vi "EOL All-Station Check Switch Signals.vi"(0 "Current Data In":sgl[][](array[numeric]), 1 "Switch Value Configuration":T3[](array[typedef])=[{"All Motions"=enum."Glass Teach", "Array"=[{"Min"=0.0, "Max"=0.0, "Check?"=FALSE}, {"Min"=0.0, "Max"=0.0, "Check?"=FALSE}, {"Min"=0.0, "Max"=0.0, "Check?"=FALSE}, {"Min"=0.0, "Max"=0.0, "Check?"=FALSE}, {"Min"=0.0, "Max"=0.0, "Check?"=FALSE}, {"Min"=0.0, "Max"=0.0, "Check?"=FALSE}, {"Min"=0.0, "Max"=0.0, "Check?"=FALSE}, {"Min"=0.0, "Max"=0.0, "Check?"=FALSE}, {"Min"=0.0, "Max"=0.0, "Check?"=FALSE}, {"Min"=0.0, "Max"=0.0, "Check?"=FALSE}, {"Min"=0.0, "Max"=0.0, "Check?"=FALSE}]}, {"All Motions"=enum."Glass Slide Open", "Array"=[{"Min"=0.0, "Max"=0.0, "Check?"=FALSE}, {"Min"=0.0, "Max"=0.0, "Check?"=FALSE}, {"Min"=0.0, "Max"=0.0, "Check?"=FALSE}, {"Min"=0.0, "Max"=0.0, "Check?"=FALSE}, {"Min"=0.0, "Max"=0.0, "Check?"=FALSE}, {"Min"=0.0, "Max"=0.0, "Check?"=FALSE}, {"Min"=0.0, "Max"=0.0, "Check?"=FALSE}, {"Min"=0.0, "Max"=0.0, "Check?"=FALSE}, {"Min"=0.0, "Max"=0.0, "Check?"=FALSE}, {"Min"=0.0, "Max"=0.0, "Check?"=FALSE}, {"Min"=0.0, "Max"=0.0, "Check?"=FALSE}]}, {"All Motions"=enum."Glass Slide Close", "Array"=[{"Min"=0.0, "Max"=0.0, "Check?"=FALSE}, {"Min"=0.0, "Max"=0.0, "Check?"=FALSE}, {"Min"=0.0, "Max"=0.0, "Check?"=FALSE}, {"Min"=0.0, "Max"=0.0, "Check?"=FALSE}, {"Min"=0.0, "Max"=0.0, "Check?"=FALSE}, {"Min"=0.0, "Max"=0.0, "Check?"=FALSE}, {"Min"=0.0, "Max"=0.0, "Check?"=FALSE}, {"Min"=0.0, "Max"=0.0, "Check?"=FALSE}, {"Min"=0.0, "Max"=0.0, "Check?"=FALSE}, {"Min"=0.0, "Max"=0.0, "Check?"=FALSE}, {"Min"=0.0, "Max"=0.0, "Check?"=FALSE}]}, {"All Motions"=enum."Glass Vent Open", "Array"=[{"Min"=0.0, "Max"=0.0, "Check?"=FALSE}, {"Min"=0.0, "Max"=0.0, "Check?"=FALSE}, {"Min"=0.0, "Max"=0.0, "Check?"=FALSE}, {"Min"=0.0, "Max"=0.0, "Check?"=FALSE}, {"Min"=0.0, "Max"=0.0, "Check?"=FALSE}, {"Min"=0.0, "Max"=0.0, "Check?"=FALSE}, {"Min"=0.0, "Max"=0.0, "Check?"=FALSE}, {"Min"=0.0, "Max"=0.0, "Check?"=FALSE}, {"Min"=0.0, "Max"=0.0, "Check?"=FALSE}, {"Min"=0.0, "Max"=0.0, "Check?"=FALSE}, {"Min"=0.0, "Max"=0.0, "Check?"=FALSE}]}, {"All Motions"=enum."Sunshade Teach", "Array"=[{"Min"=0.0, "Max"=0.0, "Check?"=FALSE}, {"Min"=0.0, "Max"=0.0, "Check?"=FALSE}, {"Min"=0.0, "Max"=0.0, "Check?"=FALSE}, {"Min"=0.0, "Max"=0.0, "Check?"=FALSE}, {"Min"=0.0, "Max"=0.0, "Check?"=FALSE}, {"Min"=0.0, "Max"=0.0, "Check?"=FALSE}, {"Min"=0.0, "Max"=0.0, "Check?"=FALSE}, {"Min"=0.0, "Max"=0.0, "Check?"=FALSE}, {"Min"=0.0, "Max"=0.0, "Check?"=FALSE}, {"Min"=0.0, "Max"=0.0, "Check?"=FALSE}, {"Min"=0.0, "Max"=0.0, "Check?"=FALSE}]}, {"All Motions"=enum."Sunshade Open", "Array"=[{"Min"=0.0, "Max"=0.0, "Check?"=FALSE}, {"Min"=0.0, "Max"=0.0, "Check?"=FALSE}, {"Min"=0.0, "Max"=0.0, "Check?"=FALSE}, {"Min"=0.0, "Max"=0.0, "Check?"=FALSE}, {"Min"=0.0, "Max"=0.0, "Check?"=FALSE}, {"Min"=0.0, "Max"=0.0, "Check?"=FALSE}, {"Min"=0.0, "Max"=0.0, "Check?"=FALSE}, {"Min"=0.0, "Max"=0.0, "Check?"=FALSE}, {"Min"=0.0, "Max"=0.0, "Check?"=FALSE}, {"Min"=0.0, "Max"=0.0, "Check?"=FALSE}, {"Min"=0.0, "Max"=0.0, "Check?"=FALSE}]}, {"All Motions"=enum."Sunshade Close", "Array"=[{"Min"=0.0, "Max"=0.0, "Check?"=FALSE}, {"Min"=0.0, "Max"=0.0, "Check?"=FALSE}, {"Min"=0.0, "Max"=0.0, "Check?"=FALSE}, {"Min"=0.0, "Max"=0.0, "Check?"=FALSE}, {"Min"=0.0, "Max"=0.0, "Check?"=FALSE}, {"Min"=0.0, "Max"=0.0, "Check?"=FALSE}, {"Min"=0.0, "Max"=0.0, "Check?"=FALSE}, {"Min"=0.0, "Max"=0.0, "Check?"=FALSE}, {"Min"=0.0, "Max"=0.0, "Check?"=FALSE}, {"Min"=0.0, "Max"=0.0, "Check?"=FALSE}, {"Min"=0.0, "Max"=0.0, "Check?"=FALSE}]}, {"All Motions"=enum."Idle", "Array"=[{"Min"=0.0, "Max"=0.0, "Check?"=FALSE}, {"Min"=0.0, "Max"=0.0, "Check?"=FALSE}, {"Min"=0.0, "Max"=0.0, "Check?"=FALSE}, {"Min"=0.0, "Max"=0.0, "Check?"=FALSE}, {"Min"=0.0, "Max"=0.0, "Check?"=FALSE}, {"Min"=0.0, "Max"=0.0, "Check?"=FALSE}, {"Min"=0.0, "Max"=0.0, "Check?"=FALSE}, {"Min"=0.0, "Max"=0.0, "Check?"=FALSE}, {"Min"=0.0, "Max"=0.0, "Check?"=FALSE}, {"Min"=0.0, "Max"=0.0, "Check?"=FALSE}, {"Min"=0.0, "Max"=0.0, "Check?"=FALSE}]}, {"All Motions"=enum."Sunshade Open 2", "Array"=[{"Min"=0.0, "Max"=0.0, "Check?"=FALSE}, {"Min"=0.0, "Max"=0.0, "Check?"=FALSE}, {"Min"=0.0, "Max"=0.0, "Check?"=FALSE}, {"Min"=0.0, "Max"=0.0, "Check?"=FALSE}, {"Min"=0.0, "Max"=0.0, "Check?"=FALSE}, {"Min"=0.0, "Max"=0.0, "Check?"=FALSE}, {"Min"=0.0, "Max"=0.0, "Check?"=FALSE}, {"Min"=0.0, "Max"=0.0, "Check?"=FALSE}, {"Min"=0.0, "Max"=0.0, "Check?"=FALSE}, {"Min"=0.0, "Max"=0.0, "Check?"=FALSE}, {"Min"=0.0, "Max"=0.0, "Check?"=FALSE}]}, {"All Motions"=enum."Sunshade Close 2", "Array"=[{"Min"=0.0, "Max"=0.0, "Check?"=FALSE}, {"Min"=0.0, "Max"=0.0, "Check?"=FALSE}, {"Min"=0.0, "Max"=0.0, "Check?"=FALSE}, {"Min"=0.0, "Max"=0.0, "Check?"=FALSE}, {"Min"=0.0, "Max"=0.0, "Check?"=FALSE}, {"Min"=0.0, "Max"=0.0, "Check?"=FALSE}, {"Min"=0.0, "Max"=0.0, "Check?"=FALSE}, {"Min"=0.0, "Max"=0.0, "Check?"=FALSE}, {"Min"=0.0, "Max"=0.0, "Check?"=FALSE}, {"Min"=0.0, "Max"=0.0, "Check?"=FALSE}, {"Min"=0.0, "Max"=0.0, "Check?"=FALSE}]}, {"All Motions"=enum."Glass Slide Open Sunshade Open", "Array"=[{"Min"=0.0, "Max"=0.0, "Check?"=FALSE}, {"Min"=0.0, "Max"=0.0, "Check?"=FALSE}, {"Min"=0.0, "Max"=0.0, "Check?"=FALSE}, {"Min"=0.0, "Max"=0.0, "Check?"=FALSE}, {"Min"=0.0, "Max"=0.0, "Check?"=FALSE}, {"Min"=0.0, "Max"=0.0, "Check?"=FALSE}, {"Min"=0.0, "Max"=0.0, "Check?"=FALSE}, {"Min"=0.0, "Max"=0.0, "Check?"=FALSE}, {"Min"=0.0, "Max"=0.0, "Check?"=FALSE}, {"Min"=0.0, "Max"=0.0, "Check?"=FALSE}, {"Min"=0.0, "Max"=0.0, "Check?"=FALSE}]}, {"All Motions"=enum."Glass Slide Open Sunshade Close", "Array"=[{"Min"=0.0, "Max"=0.0, "Check?"=FALSE}, {"Min"=0.0, "Max"=0.0, "Check?"=FALSE}, {"Min"=0.0, "Max"=0.0, "Check?"=FALSE}, {"Min"=0.0, "Max"=0.0, "Check?"=FALSE}, {"Min"=0.0, "Max"=0.0, "Check?"=FALSE}, {"Min"=0.0, "Max"=0.0, "Check?"=FALSE}, {"Min"=0.0, "Max"=0.0, "Check?"=FALSE}, {"Min"=0.0, "Max"=0.0, "Check?"=FALSE}, {"Min"=0.0, "Max"=0.0, "Check?"=FALSE}, {"Min"=0.0, "Max"=0.0, "Check?"=FALSE}, {"Min"=0.0, "Max"=0.0, "Check?"=FALSE}]}, {"All Motions"=enum."Glass Slide Close Sunshade Open", "Array"=[{"Min"=0.0, "Max"=0.0, "Check?"=FALSE}, {"Min"=0.0, "Max"=0.0, "Check?"=FALSE}, {"Min"=0.0, "Max"=0.0, "Check?"=FALSE}, {"Min"=0.0, "Max"=0.0, "Check?"=FALSE}, {"Min"=0.0, "Max"=0.0, "Check?"=FALSE}, {"Min"=0.0, "Max"=0.0, "Check?"=FALSE}, {"Min"=0.0, "Max"=0.0, "Check?"=FALSE}, {"Min"=0.0, "Max"=0.0, "Check?"=FALSE}, {"Min"=0.0, "Max"=0.0, "Check?"=FALSE}, {"Min"=0.0, "Max"=0.0, "Check?"=FALSE}, {"Min"=0.0, "Max"=0.0, "Check?"=FALSE}]}, {"All Motions"=enum."Glass Slide Close Sunshade Close", "Array"=[{"Min"=0.0, "Max"=0.0, "Check?"=FALSE}, {"Min"=0.0, "Max"=0.0, "Check?"=FALSE}, {"Min"=0.0, "Max"=0.0, "Check?"=FALSE}, {"Min"=0.0, "Max"=0.0, "Check?"=FALSE}, {"Min"=0.0, "Max"=0.0, "Check?"=FALSE}, {"Min"=0.0, "Max"=0.0, "Check?"=FALSE}, {"Min"=0.0, "Max"=0.0, "Check?"=FALSE}, {"Min"=0.0, "Max"=0.0, "Check?"=FALSE}, {"Min"=0.0, "Max"=0.0, "Check?"=FALSE}, {"Min"=0.0, "Max"=0.0, "Check?"=FALSE}, {"Min"=0.0, "Max"=0.0, "Check?"=FALSE}]}, {"All Motions"=enum."Glass Vent Open Sunshade Open", "Array"=[{"Min"=0.0, "Max"=0.0, "Check?"=FALSE}, {"Min"=0.0, "Max"=0.0, "Check?"=FALSE}, {"Min"=0.0, "Max"=0.0, "Check?"=FALSE}, {"Min"=0.0, "Max"=0.0, "Check?"=FALSE}, {"Min"=0.0, "Max"=0.0, "Check?"=FALSE}, {"Min"=0.0, "Max"=0.0, "Check?"=FALSE}, {"Min"=0.0, "Max"=0.0, "Check?"=FALSE}, {"Min"=0.0, "Max"=0.0, "Check?"=FALSE}, {"Min"=0.0, "Max"=0.0, "Check?"=FALSE}, {"Min"=0.0, "Max"=0.0, "Check?"=FALSE}, {"Min"=0.0, "Max"=0.0, "Check?"=FALSE}]}, {"All Motions"=enum."Glass Vent Open Sunshade Close", "Array"=[{"Min"=0.0, "Max"=0.0, "Check?"=FALSE}, {"Min"=0.0, "Max"=0.0, "Check?"=FALSE}, {"Min"=0.0, "Max"=0.0, "Check?"=FALSE}, {"Min"=0.0, "Max"=0.0, "Check?"=FALSE}, {"Min"=0.0, "Max"=0.0, "Check?"=FALSE}, {"Min"=0.0, "Max"=0.0, "Check?"=FALSE}, {"Min"=0.0, "Max"=0.0, "Check?"=FALSE}, {"Min"=0.0, "Max"=0.0, "Check?"=FALSE}, {"Min"=0.0, "Max"=0.0, "Check?"=FALSE}, {"Min"=0.0, "Max"=0.0, "Check?"=FALSE}, {"Min"=0.0, "Max"=0.0, "Check?"=FALSE}]}, {"All Motions"=enum."Glass Vent Close Sunshade Open", "Array"=[{"Min"=0.0, "Max"=0.0, "Check?"=FALSE}, {"Min"=0.0, "Max"=0.0, "Check?"=FALSE}, {"Min"=0.0, "Max"=0.0, "Check?"=FALSE}, {"Min"=0.0, "Max"=0.0, "Check?"=FALSE}, {"Min"=0.0, "Max"=0.0, "Check?"=FALSE}, {"Min"=0.0, "Max"=0.0, "Check?"=FALSE}, {"Min"=0.0, "Max"=0.0, "Check?"=FALSE}, {"Min"=0.0, "Max"=0.0, "Check?"=FALSE}, {"Min"=0.0, "Max"=0.0, "Check?"=FALSE}, {"Min"=0.0, "Max"=0.0, "Check?"=FALSE}, {"Min"=0.0, "Max"=0.0, "Check?"=FALSE}]}, {"All Motions"=enum."Glass Vent Close Sunshade Close", "Array"=[{"Min"=0.0, "Max"=0.0, "Check?"=FALSE}, {"Min"=0.0, "Max"=0.0, "Check?"=FALSE}, {"Min"=0.0, "Max"=0.0, "Check?"=FALSE}, {"Min"=0.0, "Max"=0.0, "Check?"=FALSE}, {"Min"=0.0, "Max"=0.0, "Check?"=FALSE}, {"Min"=0.0, "Max"=0.0, "Check?"=FALSE}, {"Min"=0.0, "Max"=0.0, "Check?"=FALSE}, {"Min"=0.0, "Max"=0.0, "Check?"=FALSE}, {"Min"=0.0, "Max"=0.0, "Check?"=FALSE}, {"Min"=0.0, "Max"=0.0, "Check?"=FALSE}, {"Min"=0.0, "Max"=0.0, "Check?"=FALSE}]}, {"All Motions"=enum."Express Glass Slide Open", "Array"=[{"Min"=0.0, "Max"=0.0, "Check?"=FALSE}, {"Min"=0.0, "Max"=0.0, "Check?"=FALSE}, {"Min"=0.0, "Max"=0.0, "Check?"=FALSE}, {"Min"=0.0, "Max"=0.0, "Check?"=FALSE}, {"Min"=0.0, "Max"=0.0, "Check?"=FALSE}, {"Min"=0.0, "Max"=0.0, "Check?"=FALSE}, {"Min"=0.0, "Max"=0.0, "Check?"=FALSE}, {"Min"=0.0, "Max"=0.0, "Check?"=FALSE}, {"Min"=0.0, "Max"=0.0, "Check?"=FALSE}, {"Min"=0.0, "Max"=0.0, "Check?"=FALSE}, {"Min"=0.0, "Max"=0.0, "Check?"=FALSE}]}, {"All Motions"=enum."Express Glass Slide Close", "Array"=[{"Min"=0.0, "Max"=0.0, "Check?"=FALSE}, {"Min"=0.0, "Max"=0.0, "Check?"=FALSE}, {"Min"=0.0, "Max"=0.0, "Check?"=FALSE}, {"Min"=0.0, "Max"=0.0, "Check?"=FALSE}, {"Min"=0.0, "Max"=0.0, "Check?"=FALSE}, {"Min"=0.0, "Max"=0.0, "Check?"=FALSE}, {"Min"=0.0, "Max"=0.0, "Check?"=FALSE}, {"Min"=0.0, "Max"=0.0, "Check?"=FALSE}, {"Min"=0.0, "Max"=0.0, "Check?"=FALSE}, {"Min"=0.0, "Max"=0.0, "Check?"=FALSE}, {"Min"=0.0, "Max"=0.0, "Check?"=FALSE}]}, {"All Motions"=enum."Express Glass Vent Open", "Array"=[{"Min"=0.0, "Max"=0.0, "Check?"=FALSE}, {"Min"=0.0, "Max"=0.0, "Check?"=FALSE}, {"Min"=0.0, "Max"=0.0, "Check?"=FALSE}, {"Min"=0.0, "Max"=0.0, "Check?"=FALSE}, {"Min"=0.0, "Max"=0.0, "Check?"=FALSE}, {"Min"=0.0, "Max"=0.0, "Check?"=FALSE}, {"Min"=0.0, "Max"=0.0, "Check?"=FALSE}, {"Min"=0.0, "Max"=0.0, "Check?"=FALSE}, {"Min"=0.0, "Max"=0.0, "Check?"=FALSE}, {"Min"=0.0, "Max"=0.0, "Check?"=FALSE}, {"Min"=0.0, "Max"=0.0, "Check?"=FALSE}]}, {"All Motions"=enum."Express Glass Vent Close", "Array"=[{"Min"=0.0, "Max"=0.0, "Check?"=FALSE}, {"Min"=0.0, "Max"=0.0, "Check?"=FALSE}, {"Min"=0.0, "Max"=0.0, "Check?"=FALSE}, {"Min"=0.0, "Max"=0.0, "Check?"=FALSE}, {"Min"=0.0, "Max"=0.0, "Check?"=FALSE}, {"Min"=0.0, "Max"=0.0, "Check?"=FALSE}, {"Min"=0.0, "Max"=0.0, "Check?"=FALSE}, {"Min"=0.0, "Max"=0.0, "Check?"=FALSE}, {"Min"=0.0, "Max"=0.0, "Check?"=FALSE}, {"Min"=0.0, "Max"=0.0, "Check?"=FALSE}, {"Min"=0.0, "Max"=0.0, "Check?"=FALSE}]}, {"All Motions"=enum."Express Sunshade Open", "Array"=[{"Min"=0.0, "Max"=0.0, "Check?"=FALSE}, {"Min"=0.0, "Max"=0.0, "Check?"=FALSE}, {"Min"=0.0, "Max"=0.0, "Check?"=FALSE}, {"Min"=0.0, "Max"=0.0, "Check?"=FALSE}, {"Min"=0.0, "Max"=0.0, "Check?"=FALSE}, {"Min"=0.0, "Max"=0.0, "Check?"=FALSE}, {"Min"=0.0, "Max"=0.0, "Check?"=FALSE}, {"Min"=0.0, "Max"=0.0, "Check?"=FALSE}, {"Min"=0.0, "Max"=0.0, "Check?"=FALSE}, {"Min"=0.0, "Max"=0.0, "Check?"=FALSE}, {"Min"=0.0, "Max"=0.0, "Check?"=FALSE}]}, {"All Motions"=enum."Express Sunshade Close", "Array"=[{"Min"=0.0, "Max"=0.0, "Check?"=FALSE}, {"Min"=0.0, "Max"=0.0, "Check?"=FALSE}, {"Min"=0.0, "Max"=0.0, "Check?"=FALSE}, {"Min"=0.0, "Max"=0.0, "Check?"=FALSE}, {"Min"=0.0, "Max"=0.0, "Check?"=FALSE}, {"Min"=0.0, "Max"=0.0, "Check?"=FALSE}, {"Min"=0.0, "Max"=0.0, "Check?"=FALSE}, {"Min"=0.0, "Max"=0.0, "Check?"=FALSE}, {"Min"=0.0, "Max"=0.0, "Check?"=FALSE}, {"Min"=0.0, "Max"=0.0, "Check?"=FALSE}, {"Min"=0.0, "Max"=0.0, "Check?"=FALSE}]}, {"All Motions"=enum."Express Sunshade Open 2", "Array"=[{"Min"=0.0, "Max"=0.0, "Check?"=FALSE}, {"Min"=0.0, "Max"=0.0, "Check?"=FALSE}, {"Min"=0.0, "Max"=0.0, "Check?"=FALSE}, {"Min"=0.0, "Max"=0.0, "Check?"=FALSE}, {"Min"=0.0, "Max"=0.0, "Check?"=FALSE}, {"Min"=0.0, "Max"=0.0, "Check?"=FALSE}, {"Min"=0.0, "Max"=0.0, "Check?"=FALSE}, {"Min"=0.0, "Max"=0.0, "Check?"=FALSE}, {"Min"=0.0, "Max"=0.0, "Check?"=FALSE}, {"Min"=0.0, "Max"=0.0, "Check?"=FALSE}, {"Min"=0.0, "Max"=0.0, "Check?"=FALSE}]}, {"All Motions"=enum."Express Sunshade Close 2", "Array"=[{"Min"=0.0, "Max"=0.0, "Check?"=FALSE}, {"Min"=0.0, "Max"=0.0, "Check?"=FALSE}, {"Min"=0.0, "Max"=0.0, "Check?"=FALSE}, {"Min"=0.0, "Max"=0.0, "Check?"=FALSE}, {"Min"=0.0, "Max"=0.0, "Check?"=FALSE}, {"Min"=0.0, "Max"=0.0, "Check?"=FALSE}, {"Min"=0.0, "Max"=0.0, "Check?"=FALSE}, {"Min"=0.0, "Max"=0.0, "Check?"=FALSE}, {"Min"=0.0, "Max"=0.0, "Check?"=FALSE}, {"Min"=0.0, "Max"=0.0, "Check?"=FALSE}, {"Min"=0.0, "Max"=0.0, "Check?"=FALSE}]}, {"All Motions"=enum."Express Glass Slide Open Sunshade Open", "Array"=[{"Min"=0.0, "Max"=0.0, "Check?"=FALSE}, {"Min"=0.0, "Max"=0.0, "Check?"=FALSE}, {"Min"=0.0, "Max"=0.0, "Check?"=FALSE}, {"Min"=0.0, "Max"=0.0, "Check?"=FALSE}, {"Min"=0.0, "Max"=0.0, "Check?"=FALSE}, {"Min"=0.0, "Max"=0.0, "Check?"=FALSE}, {"Min"=0.0, "Max"=0.0, "Check?"=FALSE}, {"Min"=0.0, "Max"=0.0, "Check?"=FALSE}, {"Min"=0.0, "Max"=0.0, "Check?"=FALSE}, {"Min"=0.0, "Max"=0.0, "Check?"=FALSE}, {"Min"=0.0, "Max"=0.0, "Check?"=FALSE}]}, {"All Motions"=enum."Express Glass Slide Open Sunshade Close", "Array"=[{"Min"=0.0, "Max"=0.0, "Check?"=FALSE}, {"Min"=0.0, "Max"=0.0, "Check?"=FALSE}, {"Min"=0.0, "Max"=0.0, "Check?"=FALSE}, {"Min"=0.0, "Max"=0.0, "Check?"=FALSE}, {"Min"=0.0, "Max"=0.0, "Check?"=FALSE}, {"Min"=0.0, "Max"=0.0, "Check?"=FALSE}, {"Min"=0.0, "Max"=0.0, "Check?"=FALSE}, {"Min"=0.0, "Max"=0.0, "Check?"=FALSE}, {"Min"=0.0, "Max"=0.0, "Check?"=FALSE}, {"Min"=0.0, "Max"=0.0, "Check?"=FALSE}, {"Min"=0.0, "Max"=0.0, "Check?"=FALSE}]}, {"All Motions"=enum."Express Glass Slide Close Sunshade Open", "Array"=[{"Min"=0.0, "Max"=0.0, "Check?"=FALSE}, {"Min"=0.0, "Max"=0.0, "Check?"=FALSE}, {"Min"=0.0, "Max"=0.0, "Check?"=FALSE}, {"Min"=0.0, "Max"=0.0, "Check?"=FALSE}, {"Min"=0.0, "Max"=0.0, "Check?"=FALSE}, {"Min"=0.0, "Max"=0.0, "Check?"=FALSE}, {"Min"=0.0, "Max"=0.0, "Check?"=FALSE}, {"Min"=0.0, "Max"=0.0, "Check?"=FALSE}, {"Min"=0.0, "Max"=0.0, "Check?"=FALSE}, {"Min"=0.0, "Max"=0.0, "Check?"=FALSE}, {"Min"=0.0, "Max"=0.0, "Check?"=FALSE}]}, {"All Motions"=enum."Express Glass Slide Close Sunshade Close", "Array"=[{"Min"=0.0, "Max"=0.0, "Check?"=FALSE}, {"Min"=0.0, "Max"=0.0, "Check?"=FALSE}, {"Min"=0.0, "Max"=0.0, "Check?"=FALSE}, {"Min"=0.0, "Max"=0.0, "Check?"=FALSE}, {"Min"=0.0, "Max"=0.0, "Check?"=FALSE}, {"Min"=0.0, "Max"=0.0, "Check?"=FALSE}, {"Min"=0.0, "Max"=0.0, "Check?"=FALSE}, {"Min"=0.0, "Max"=0.0, "Check?"=FALSE}, {"Min"=0.0, "Max"=0.0, "Check?"=FALSE}, {"Min"=0.0, "Max"=0.0, "Check?"=FALSE}, {"Min"=0.0, "Max"=0.0, "Check?"=FALSE}]}, {"All Motions"=enum."Express Glass Vent Open Sunshade Open", "Array"=[{"Min"=0.0, "Max"=0.0, "Check?"=FALSE}, {"Min"=0.0, "Max"=0.0, "Check?"=FALSE}, {"Min"=0.0, "Max"=0.0, "Check?"=FALSE}, {"Min"=0.0, "Max"=0.0, "Check?"=FALSE}, {"Min"=0.0, "Max"=0.0, "Check?"=FALSE}, {"Min"=0.0, "Max"=0.0, "Check?"=FALSE}, {"Min"=0.0, "Max"=0.0, "Check?"=FALSE}, {"Min"=0.0, "Max"=0.0, "Check?"=FALSE}, {"Min"=0.0, "Max"=0.0, "Check?"=FALSE}, {"Min"=0.0, "Max"=0.0, "Check?"=FALSE}, {"Min"=0.0, "Max"=0.0, "Check?"=FALSE}]}, {"All Motions"=enum."Express Glass Vent Open Sunshade Close", "Array"=[{"Min"=0.0, "Max"=0.0, "Check?"=FALSE}, {"Min"=0.0, "Max"=0.0, "Check?"=FALSE}, {"Min"=0.0, "Max"=0.0, "Check?"=FALSE}, {"Min"=0.0, "Max"=0.0, "Check?"=FALSE}, {"Min"=0.0, "Max"=0.0, "Check?"=FALSE}, {"Min"=0.0, "Max"=0.0, "Check?"=FALSE}, {"Min"=0.0, "Max"=0.0, "Check?"=FALSE}, {"Min"=0.0, "Max"=0.0, "Check?"=FALSE}, {"Min"=0.0, "Max"=0.0, "Check?"=FALSE}, {"Min"=0.0, "Max"=0.0, "Check?"=FALSE}, {"Min"=0.0, "Max"=0.0, "Check?"=FALSE}]}, {"All Motions"=enum."Express Glass Vent Close Sunshade Open", "Array"=[{"Min"=0.0, "Max"=0.0, "Check?"=FALSE}, {"Min"=0.0, "Max"=0.0, "Check?"=FALSE}, {"Min"=0.0, "Max"=0.0, "Check?"=FALSE}, {"Min"=0.0, "Max"=0.0, "Check?"=FALSE}, {"Min"=0.0, "Max"=0.0, "Check?"=FALSE}, {"Min"=0.0, "Max"=0.0, "Check?"=FALSE}, {"Min"=0.0, "Max"=0.0, "Check?"=FALSE}, {"Min"=0.0, "Max"=0.0, "Check?"=FALSE}, {"Min"=0.0, "Max"=0.0, "Check?"=FALSE}, {"Min"=0.0, "Max"=0.0, "Check?"=FALSE}, {"Min"=0.0, "Max"=0.0, "Check?"=FALSE}]}, {"All Motions"=enum."Express Glass Vent Close Sunshade Close", "Array"=[{"Min"=0.0, "Max"=0.0, "Check?"=FALSE}, {"Min"=0.0, "Max"=0.0, "Check?"=FALSE}, {"Min"=0.0, "Max"=0.0, "Check?"=FALSE}, {"Min"=0.0, "Max"=0.0, "Check?"=FALSE}, {"Min"=0.0, "Max"=0.0, "Check?"=FALSE}, {"Min"=0.0, "Max"=0.0, "Check?"=FALSE}, {"Min"=0.0, "Max"=0.0, "Check?"=FALSE}, {"Min"=0.0, "Max"=0.0, "Check?"=FALSE}, {"Min"=0.0, "Max"=0.0, "Check?"=FALSE}, {"Min"=0.0, "Max"=0.0, "Check?"=FALSE}, {"Min"=0.0, "Max"=0.0, "Check?"=FALSE}]}], 3 "Communication Type":T2, 5 "Current Data Index In":i32, 7 "Motion":T1, 9 "Check Switch Signals":T1, 11 "Error Table In":string[][](table), 12 "station idx":i32=4) -> (4 "Current Data Out":sgl[][](array[numeric]), 6 "Current Data Index Out":i32, 10 "Pass?":bool, 14 "Switches 1 to 8":dbl[](array[numeric]), 15 "Error Table Out":string[][](array[string]))   [LabVIEW 2018]
uses:
  02.Type Def's/All Motions.ctl
  02.Type Def's/EOL Switch Value Configuration Cluster.ctl
  02.Type Def's/EOL Switch Max Min Check Cluster.ctl
  02.Type Def's/All Communication Types.ctl
  02.Type Def's/EOL Analog Input Control.ctl
panel:
  # "Min"
  # "Max"
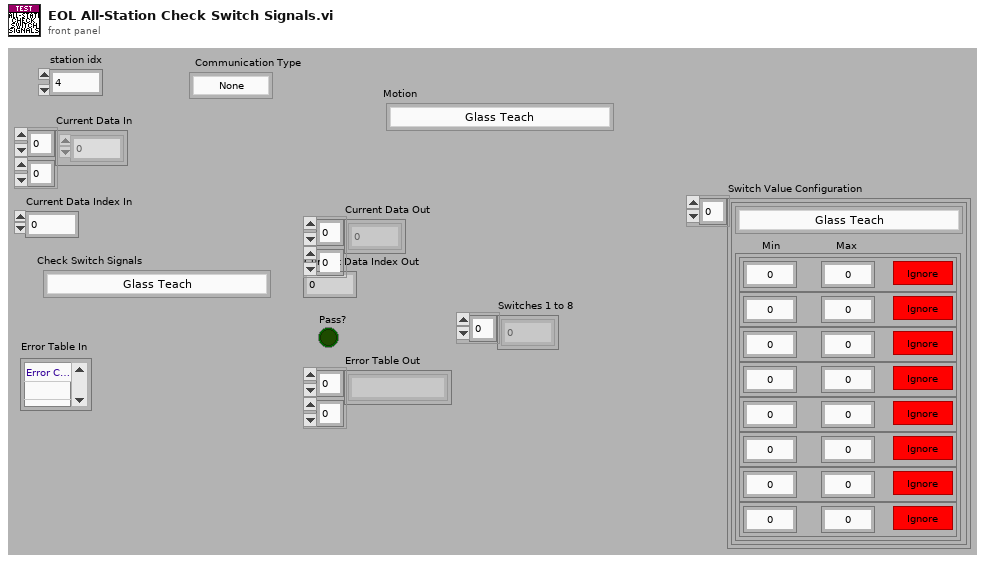
[diagram p1: front panel]
types:
  T1 = typedef "All Motions.ctl" = enum16{"Glass Teach", "Glass Slide Open", "Glass Slide Close", "Glass Vent Open", "Glass Vent Close", "Sunshade Teach", "Sunshade Open", "Sunshade Close", "Idle", "Sunshade Open 2", "Sunshade Close 2", "Glass Slide Open Sunshade Open", "Glass Slide Open Sunshade Close", "Glass Slide Close Sunshade Open", "Glass Slide Close Sunshade Close", "Glass Vent Open Sunshade Open", "Glass Vent Open Sunshade Close", "Glass Vent Close Sunshade Open", "Glass Vent Close Sunshade Close", "Express Glass Slide Open", "Express Glass Slide Close", "Express Glass Vent Open", "Express Glass Vent Close", "Express Sunshade Open", "Express Sunshade Close", "Express Sunshade Open 2", "Express Sunshade Close 2", "Express Glass Slide Open Sunshade Open", "Express Glass Slide Open Sunshade Close", "Express Glass Slide Close Sunshade Open", "Express Glass Slide Close Sunshade Close", "Express Glass Vent Open Sunshade Open", "Express Glass Vent Open Sunshade Close", "Express Glass Vent Close Sunshade Open", "Express Glass Vent Close Sunshade Close", "Goto Position Glass", "Goto Position Sunshade", "Sunshade Teach 2"}
  T2 = typedef "All Communication Types.ctl" = enum16{"None", "CAN", "RS 232", "RS 232 LIN", "GM LIN", "SnT LIN", "K Line", "Robel CAN", "P42M-Continental", "Inalfa SCU LIN", "Spare 3"}
  T3 = typedef "EOL Switch Value Configuration Cluster.ctl" = cluster{"All Motions":T1, "Array":T4[]}
  T4 = typedef "EOL Switch Max Min Check Cluster.ctl" = cluster{"Min":dbl, "Max":dbl, "Check?":bool}
  T5 = typedef "EOL Analog Input Control.ctl" = enum16{"SW PS  Volage", "Switch A", "Switch B", "Switch C", "Motor Voltage", "Motor Current", "ATS"}
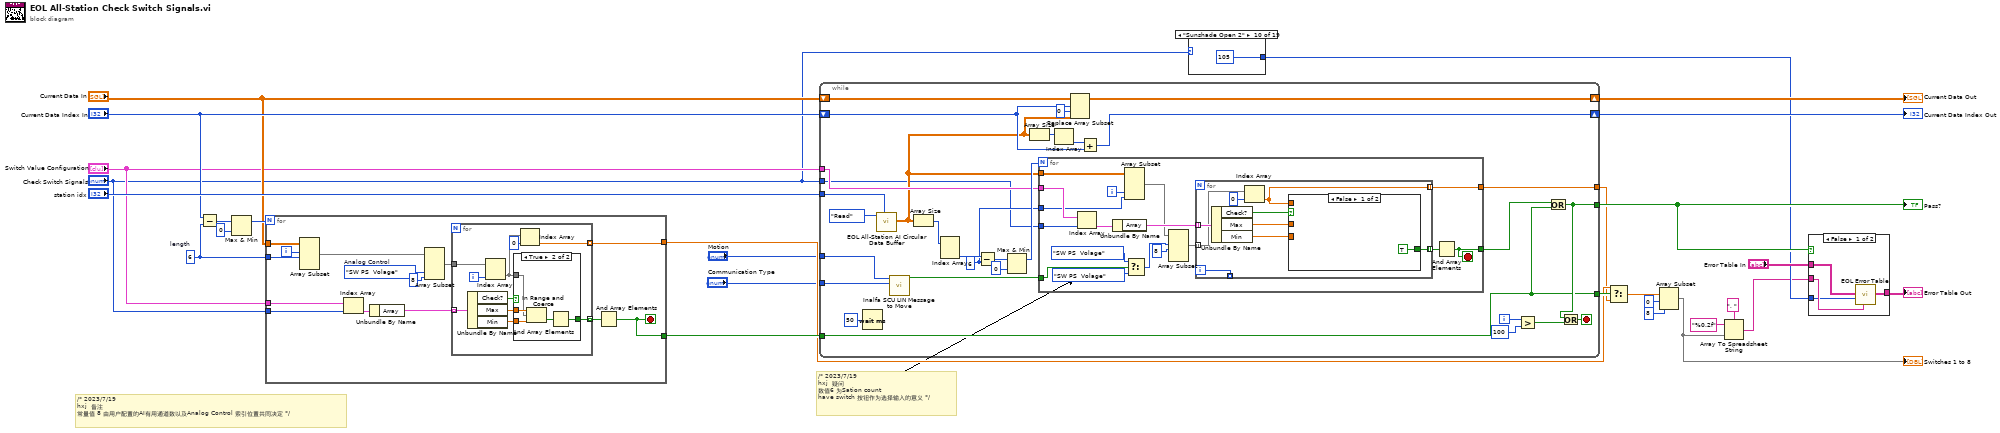
[diagram p0: block diagram]
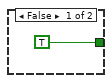
[diagram p2: hidden frame]
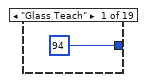
[diagram p3: hidden frame]
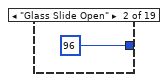
[diagram p4: hidden frame]
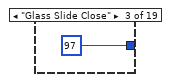
[diagram p5: hidden frame]
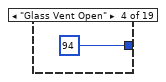
[diagram p6: hidden frame]
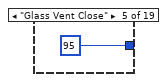
[diagram p7: hidden frame]
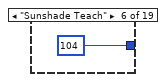
[diagram p8: hidden frame]
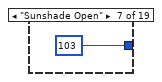
[diagram p9: hidden frame]
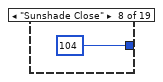
[diagram p10: hidden frame]
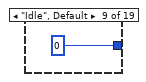
[diagram p11: hidden frame]
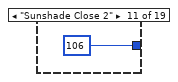
[diagram p12: hidden frame]
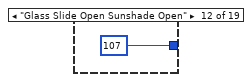
[diagram p13: hidden frame]
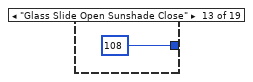
[diagram p14: hidden frame]
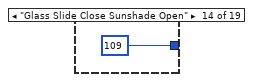
[diagram p15: hidden frame]
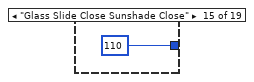
[diagram p16: hidden frame]
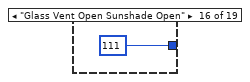
[diagram p17: hidden frame]
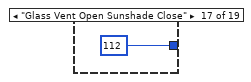
[diagram p18: hidden frame]
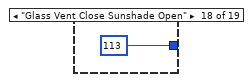
[diagram p19: hidden frame]
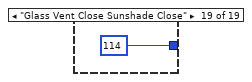
[diagram p20: hidden frame]
diagram:
  w12 = 6  # length
  # "/* 2023/7/19\nhxj  疑问\n数值6 为Sation count\nhave switch 按钮作为选择输入的意义 */"
  # "/* 2023/7/19\nhxj  备注\n常量值 8 由用户配置的AI有用通道数以及Analog Control 索引位置共同决定 */"
  n1 = Subtract(x="Current Data Index In", y=w12) -> (x-y=w18:i32)
  n2 = Max & Min(x=w18, y=0) -> (max(x,y)=w15:i32)  [unwired: 1 out]
  n3 = for {
    N: w15 -> [_]
    tunnel: "Current Data In" -> [w41]
    tunnel: "Switch Value Configuration" -> [w42]
    tunnel: w12 -> [w40]
    tunnel: "Check Switch Signals" -> [w37]
    tunnel: [w30] -> w10
    tunnel: [w29] -> w8
    i -> [w39]
    stop <- w30 stop-if-true
    w32 = EOL_Analog_Input_Control."SW PS  Volage"  # Analog Control
    n4 = Array Subset(array=w41, index (row)=w39, length (row)=w40) -> (w38:sgl[][])  [unwired: 2 in]
    n5 = Index Array(array=w42, index=w37) -> (element=w36:T3)
    n6 = Unbundle By Name(w36) -> ("Array"=w35:T4[])
    n7 = Array Subset(array=w38, index (col)=w32, length (col)=8 ("length")) -> (w34:sgl[][])  [unwired: 2 in]
    n8 = for {
      tunnel: w35 -> [w52] mode=indexing
      tunnel: w34 -> [w47]
      tunnel: [w48] -> w33 mode=indexing
      tunnel: [w43] -> w29 mode=indexing
      i -> [w46]
      n9 = Unbundle By Name(w52) -> ("Check?"=w51:bool, "Max"=w50:dbl, "Min"=w49:dbl)
      n10 = Index Array(array=w47, index (col)=w46) -> (element=w45:sgl[])  [unwired: 1 in]
      n11 = case shown="True" w51 {
        tunnel: w45 -> [_ w54]
        tunnel: w50 -> [_ w58]
        tunnel: w49 -> [_ w57]
        tunnel: [TRUE w55] -> w48
        frame False {
        }
        frame True {
          n12 = In Range and Coerce(upper limit=w58, x=w54, lower limit=w57) -> (In Range?=w56:bool[])  [unwired: 1 out]
          n13 = And Array Elements(Boolean array=w56) -> (logical AND=w55:bool)
        }
      }
      n14 = Index Array(array=w45, index=0) -> (element=w43:sgl)
    }
    n15 = And Array Elements(Boolean array=w33) -> (logical AND=w30:bool)
  }
  n16 = while {
    tunnel: [w73] -> w26
    tunnel: "Check Switch Signals" -> [w62]
    shift-right: [w78] -> w27
    shift-left: "Current Data Index In" -> [w81]
    shift-right: [w79] -> w28
    shift-left: "Current Data In" -> [w80]
    tunnel: "Switch Value Configuration" -> [w66]
    tunnel: "station idx" -> [w76]
    tunnel: w10 -> [w72]
    tunnel: [w72] -> w9
    tunnel: [w64] -> w3
    tunnel: "Communication Type" -> [w61]
    tunnel: "Motion" -> [w59]
    i -> [w86]
    stop <- w84 stop-if-true
    w67 = 6 ("y")
    n17 = Wait (ms)(milliseconds to wait=u32 50) -> ()  [unwired: 1 out]
    n18 = call "EOL All-Station AI Circular Data Buffer.vi"("station idx"=w76, "Mode"=enum16{"Initialize", "Read", "Write"}."Read") -> ("Data Read (Samp-Ro, Ch-Col)"=w65:sgl[][])  [unwired: 9 in]
    n19 = call "Inalfa SCU LIN Message to Move.vi"("Communication Type"=w61, "Motion"=w59) -> ("Have Swtich?"=w60:bool)  [unwired: 9 in]
    n20 = Array Size(array=w65) -> (size(s)=w88:i32[])
    n21 = Index Array(array=w88) -> (element #2=w69:i32)  [unwired: 2 in, 1 out]
    n22 = Subtract(x=w69, y=w67) -> (x-y=w70:i32)
    n23 = Max & Min(x=w70, y=0) -> (max(x,y)=w68:i32)  [unwired: 1 out]
    n24 = Array Size(array=w65) -> (size(s)=w82:i32[])
    n25 = for {
      N: w68 -> [_]
      tunnel: w62 -> [w105]
      tunnel: w66 -> [w104]
      tunnel: [w100] -> w63
      tunnel: w65 -> [w97]
      tunnel: w67 -> [w98]
      tunnel: [w95] -> w64
      tunnel: w60 -> [w90]
      i -> [w99]
      stop <- w100 stop-if-true
      n26 = Index Array(array=w104, index=w105) -> (element=w103:T3)
      n27 = Unbundle By Name(w103) -> ("Array"=w102:T4[])
      n28 = Array Subset(array=w97, index (col)=w99, length (col)=w98) -> (w96:sgl[][])  [unwired: 2 in]
      n29 = Select(t=EOL_Analog_Input_Control."SW PS  Volage" ("Analog Control"), s=w90, f=EOL_Analog_Input_Control."SW PS  Volage" ("Analog Control")) -> (s? t:f=w89:T5)
      n30 = Array Subset(array=w96, index (row)=w89, length (row)=8 ("length")) -> (w94:sgl[][])  [unwired: 2 in]
      n31 = for {
        tunnel: w102 -> [w114] mode=indexing
        tunnel: w94 -> [w108] mode=indexing
        tunnel: [w110] -> w101 mode=indexing
        tunnel: [w107] -> w95 mode=indexing
        tunnel: [w106] -> _ mode=indexing
        i -> [w106]
        n32 = Unbundle By Name(w114) -> ("Check?"=w113:bool, "Max"=w112:dbl, "Min"=w111:dbl)
        n33 = Index Array(array=w108, index=0) -> (element=w107:sgl)
        n34 = case shown="False" w113 {
          tunnel: w112 -> [_ w119]
          tunnel: w111 -> [_ w118]
          tunnel: [TRUE w116] -> w110
          tunnel: w107 -> [_ w117]
          frame False {
          }
          frame True {
            n35 = In Range and Coerce(upper limit=w119, x=w117, lower limit=w118) -> (In Range?=w116:bool)  [unwired: 1 out]
          }
        }
      }
      n36 = And Array Elements(Boolean array=w101) -> (logical AND=w100:bool)
    }
    n37 = Index Array(array=w82) -> (element=w74:i32)  [unwired: 1 in]
    n38 = Replace Array Subset(array=w80, new element=w65, index (row)=w81, index (col)=0 ("disabled index (col)")) -> (w79:sgl[][])
    n39 = Add(x=w74, y=w81) -> (x+y=w78:i32)
    n40 = Greater?(x=w86, y=100) -> (0:w83:bool)
    n41 = Or(x=w63, y=w72) -> (x .or. y?=w73:bool)
    n42 = Or(x=w73, y=w83) -> (x .or. y?=w84:bool)
  }
  "Pass?" <- w26
  "Current Data Index Out" <- w27
  "Current Data Out" <- w28
  n43 = case shown="\"Sunshade Open 2\"" "Check Switch Signals" {
    tunnel: [u16 94 ("Error No.") u16 96 ("Error No.") u16 97 ("Error No.") u16 94 ("Error No.") u16 95 ("Error No.") u16 104 ("Error No.") u16 103 ("Error No.") u16 104 ("Error No.") u16 0 ("Error No.") u16 105 ("Error No.") u16 106 ("Error No.") u16 107 ("Error No.") u16 108 ("Error No.") u16 109 ("Error No.") u16 110 ("Error No.") u16 111 ("Error No.") u16 112 ("Error No.") u16 113 ("Error No.") u16 114 ("Error No.")] -> w23
    frame "Glass Teach" {
    }
    frame "Glass Slide Open" {
    }
    frame "Glass Slide Close" {
    }
    frame "Glass Vent Open" {
    }
    frame "Glass Vent Close" {
    }
    frame "Sunshade Teach" {
    }
    frame "Sunshade Open" {
    }
    frame "Sunshade Close" {
    }
    frame "Idle", Default {
    }
    frame "Sunshade Open 2" {
    }
    frame "Sunshade Close 2" {
    }
    frame "Glass Slide Open Sunshade Open" {
    }
    frame "Glass Slide Open Sunshade Close" {
    }
    frame "Glass Slide Close Sunshade Open" {
    }
    frame "Glass Slide Close Sunshade Close" {
    }
    frame "Glass Vent Open Sunshade Open" {
    }
    frame "Glass Vent Open Sunshade Close" {
    }
    frame "Glass Vent Close Sunshade Open" {
    }
    frame "Glass Vent Close Sunshade Close" {
    }
  }
  n44 = Select(t=w8, s=w9, f=w3) -> (s? t:f=w7:sgl[])
  n45 = Array Subset(array=w7, index=0, length=8) -> (w6:sgl[])
  "Switches 1 to 8" <- w6
  n46 = Array To Spreadsheet String(delimiter (Tab)=", ", array=w6, 3:"%0.2f" ("format string")) -> (spreadsheet string=w20:string)
  n47 = case shown="False" w26 {
    tunnel: "Error Table In" -> [w142 w143]
    tunnel: [w139 w143] -> w24
    tunnel: w20 -> [w141 _]
    tunnel: w23 -> [w140 _]
    frame False {
      n48 = call "EOL Error Table.vi"("Error Description"=w141, "Error No."=w140, "Error Table In"=w142) -> ("Error Table Out"=w139:string[][])  [unwired: 7 in, 1 out]
    }
    frame True {
    }
  }
  "Error Table Out" <- w24
